vi "Count.vi"(8 "error in":errorcluster, 11 "Driver path":path) -> (0 "error out":errorcluster, 3 "Count":i32)   [LabVIEW 2020, in "r307-python-labview-driver.lvlib"]
uses:
  r307-python-labview-driver.lvlib
  <vilib>/Utility/error.llb/whitespace.ctl
panel:
  out "command line":string="cmc /c python \"%s\" ENROLL"
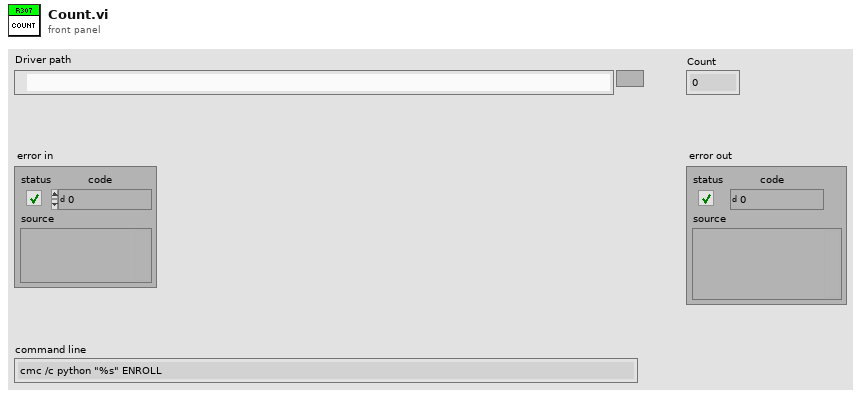
[diagram p1: front panel]
types:
  T1 = typedef "whitespace.ctl" = u16
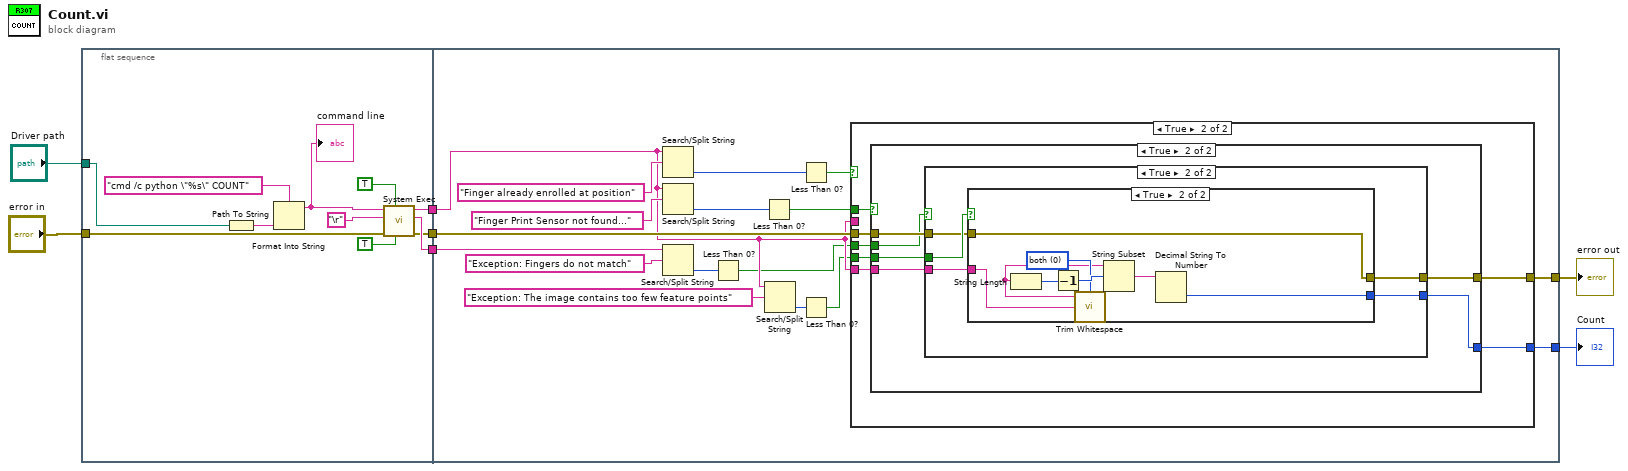
[diagram p0: block diagram]
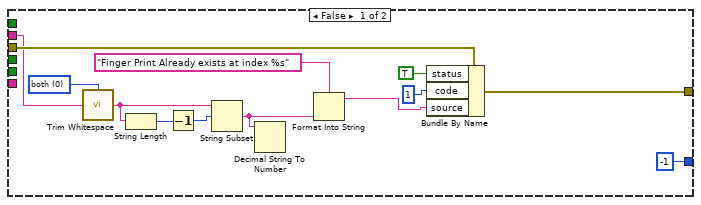
[diagram p2: hidden frame]
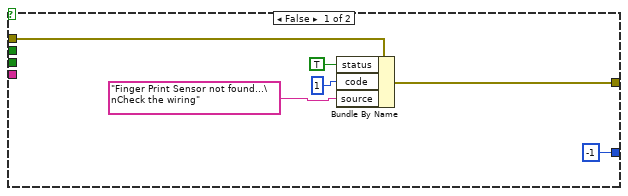
[diagram p3: hidden frame]
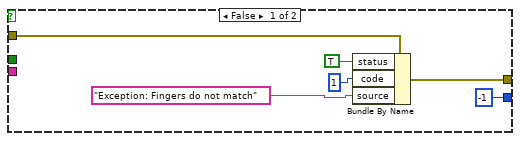
[diagram p4: hidden frame]
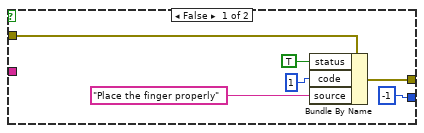
[diagram p5: hidden frame]
diagram:
  n1 = flat-sequence {
    tunnel: "Driver path" -> [w16]
    tunnel: "error in" -> [w9]
    tunnel: [w12] -> w5
    tunnel: [w8] -> w4
    tunnel: [w11] -> w3
    tunnel: w5 -> [w34]
    tunnel: w4 -> [w33]
    tunnel: w3 -> [w21]
    tunnel: [w27] -> w2
    tunnel: [w25] -> w1
    frame #0 {
      n2 = Path To String(path=w16) -> (string=w14:string)
      n3 = Format Into String(format string="cmd /c python \"%s\" COUNT" ("command line"), w14) -> (resulting string=w15:string)  [unwired: 2 in, 1 out]
      "command line" <- w15
      n4 = call <vilib>:"System Exec.vi"("run minimized? (F)"=TRUE, "wait until completion? (T)"=TRUE, "error in (no error)"=w9, "standard input"="\r", "command line"=w15) -> ("error out"=w8:errorcluster, "standard error"=w12:string, "standard output"=w11:string)  [unwired: 3 in, 1 out]
    }
    frame #1 {
      n5 = Search/Split String(string=w21, search string/char (-)="Finger already enrolled at position") -> (offset of match=w23:i32)  [unwired: 1 in, 2 out]
      n6 = Search/Split String(string=w21, search string/char (-)="Finger Print Sensor not found...") -> (offset of match=w31:i32)  [unwired: 1 in, 2 out]
      n7 = Search/Split String(string=w34, search string/char (-)="Exception: Fingers do not match") -> (offset of match=w35:i32)  [unwired: 1 in, 2 out]
      n8 = Less Than 0?(x=w35) -> (x < 0?=w20:bool)
      n9 = Less Than 0?(x=w31) -> (x < 0?=w30:bool)
      n10 = Search/Split String(string=w21, search string/char (-)="Exception: The image contains too few feature points" ("string")) -> (offset of match=w29:i32)  [unwired: 1 in, 2 out]
      n11 = Less Than 0?(x=w23) -> (x < 0?=w22:bool)
      n12 = Less Than 0?(x=w29) -> (x < 0?=w19:bool)
      n13 = case shown="True" w22 {
        tunnel: w33 -> [w46 w55]
        tunnel: w30 -> [_ w54]
        tunnel: [w43 w53] -> w27
        tunnel: w21 -> [_ w52]
        tunnel: [-1 ("Enrolled ID") w51] -> w25
        tunnel: w21 -> [w39 _]
        tunnel: w20 -> [_ w50]
        tunnel: w19 -> [_ w49]
        frame False {
          w40 = T1 0 items=["both", "start of string", "end of string"] ("location (both)")
          n14 = call <vilib>:"Trim Whitespace.vi"("string"=w39, "location (both)"=w40) -> ("trimmed string"=w36:string)
          n15 = String Length(string=w36) -> (length=w38:i32)
          n16 = Decrement(x=w38) -> (x-1=w37:i32)
          n17 = String Subset(string=w36, offset (0)=w37) -> (substring=w41:string)  [unwired: 1 in]
          n18 = Decimal String To Number(string=w41) -> ()  [unwired: 2 in, 2 out]
          n19 = Format Into String(format string="Finger Print Already exists at index %s" ("source"), w41) -> (resulting string=w44:string)  [unwired: 2 in, 1 out]
          n20 = Bundle By Name(cluster=w46, "status"=TRUE, "code"=1, "source"=w44) -> (w43:errorcluster)
        }
        frame True {
          n21 = case shown="True" w54 {
            tunnel: w55 -> [w58 w67]
            tunnel: w52 -> [_ w65]
            tunnel: [w57 w66] -> w53
            tunnel: [-1 ("Enrolled ID") w64] -> w51
            tunnel: w50 -> [_ w63]
            tunnel: w49 -> [_ w62]
            frame False {
              n22 = Bundle By Name(cluster=w58, "status"=TRUE, "code"=1, "source"="Finger Print Sensor not found...\nCheck the wiring" ("search string/char (-)")) -> (w57:errorcluster)
            }
            frame True {
              n23 = case shown="True" w63 {
                tunnel: w67 -> [w73 w75]
                tunnel: [w70 w74] -> w66
                tunnel: w65 -> [_ w78]
                tunnel: [-1 ("Enrolled ID") w77] -> w64
                tunnel: w62 -> [_ w76]
                frame False {
                  n24 = Bundle By Name(cluster=w73, "status"=TRUE, "code"=1, "source"="Exception: Fingers do not match" ("search string/char (-)")) -> (w70:errorcluster)
                }
                frame True {
                  n25 = case shown="True" w76 {
                    tunnel: w78 -> [_ w87]
                    tunnel: [-1 w91] -> w77
                    tunnel: w75 -> [w81 w88]
                    tunnel: [w80 w88] -> w74
                    frame False {
                      n26 = Bundle By Name(cluster=w81, "status"=TRUE, "code"=1, "source"="Place the finger properly" ("string")) -> (w80:errorcluster)
                    }
                    frame True {
                      w86 = T1 0 items=["both", "start of string", "end of string"] ("location (both)")
                      n27 = call <vilib>:"Trim Whitespace.vi"("string"=w87, "location (both)"=w86) -> ("trimmed string"=w85:string)
                      n28 = String Length(string=w85) -> (length=w90:i32)
                      n29 = Decrement(x=w90) -> (x-1=w89:i32)
                      n30 = String Subset(string=w85, offset (0)=w89) -> (substring=w92:string)  [unwired: 1 in]
                      n31 = Decimal String To Number(string=w92) -> (number=w91:i32)  [unwired: 2 in, 1 out]
                    }
                  }
                }
              }
            }
          }
        }
      }
    }
  }
  "error out" <- w2
  "Count" <- w1
